vi "acquire_and_wait.vi"(8 "Error in (no error)":errorcluster, 11 "stop now":refnum<vi>) -> (0 "Error out":errorcluster)   [LabVIEW 2020]
uses:
  <userlib>/caLab/Private/Put_I32_PV.vi
  <userlib>/caLab/Private/Get_PV.vi
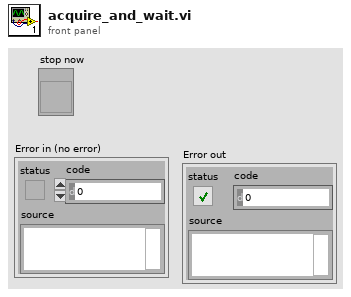
[diagram p1: front panel]
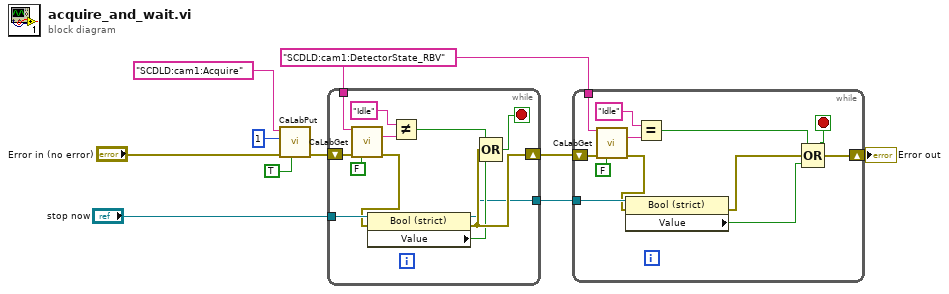
[diagram p0: block diagram]
diagram:
  w5 = "SCDLD:cam1:DetectorState_RBV"
  n1 = call-poly <userlib>:"CaLabPut.vi"("Synchronous (F)"=TRUE, "Error in (no error)"="Error in (no error)", "Value"=1 ("Numeric"), "PV Name"="SCDLD:cam1:Acquire") -> ("Error out"=w9:errorcluster)  [unwired: 4 in, 3 out]
  n2 = while {
    shift-right: [w13] -> w6
    shift-left: w9 -> [w22]
    tunnel: w5 -> [w21]
    tunnel: "stop now" -> [w15]
    tunnel: [w11] -> w1
    stop <- w16 stop-if-true
    n3 = call-poly <userlib>:"CaLabGet.vi"("PV Name"=w21, "Error in (no error)"=w22, "NoMDEL(F)"=FALSE) -> ("1rst Value (string)"=w20:string, "Error out"=w14:errorcluster)  [unwired: 6 in, 5 out]
    n4 = property class="Bool (strict)"(reference=w15, error in=w14) -> (reference out=w11:refnum<vi>, error out=w13:errorcluster, "Value"=w12:bool)
    n5 = Not Equal?(x="Idle", y=w20) -> (x != y?=w17:bool)
    n6 = Compound Arithmetic op=OR(w17, w13, w12) -> (w16:bool)
  }
  n7 = while {
    shift-right: [w24] -> w4
    shift-left: w6 -> [w33]
    tunnel: w5 -> [w32]
    tunnel: w1 -> [w26]
    stop <- w27 stop-if-true
    n8 = call-poly <userlib>:"CaLabGet.vi"("PV Name"=w32, "Error in (no error)"=w33, "NoMDEL(F)"=FALSE) -> ("1rst Value (string)"=w31:string, "Error out"=w25:errorcluster)  [unwired: 6 in, 5 out]
    n9 = property class="Bool (strict)"(reference=w26, error in=w25) -> (error out=w24:errorcluster, "Value"=w23:bool)  [unwired: 1 out]
    n10 = Equal?(x="Idle", y=w31) -> (x = y?=w28:bool)
    n11 = Compound Arithmetic op=OR(w28, w24, w23) -> (w27:bool)
  }
  "Error out" <- w4
